vi "From Pair.vi"(0 "Pair":refnum<class "Pair.lvclass">) -> (2 "Map":refnum<class "Map.lvclass">)   [LabVIEW 2018, in "Toolkit.lvlib" / "Data.lvlib" / "Map.lvclass"]
uses:
  Map.lvclass
  Pair/Pair.lvclass
  Map.lvclass/Map.ctl
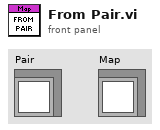
[diagram p1: front panel]
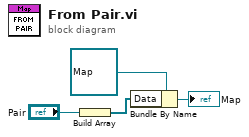
[diagram p0: block diagram]
diagram:
  n1 = Build Array("Pair") -> (w2:refnum<class "Pair.lvclass">[])
  n2 = Bundle By Name(cluster=refnum<class "Map.lvclass"> refnum ("Toolkit.lvlib:Data.lvlib:Map.lvclass"), "Data"=w2) -> (→"Map":refnum<class "Map.lvclass">)
